vi "Modify Window Style.vi"(7 "Style Value":bool, 8 "GWL_EXStyle Modify":T1(ring), 9 "GWL_EXStyle In":u32 format="%.0x", 10 "GWL_Style Modify":T2(ring), 11 "GWL_Style In":u32 format="%.0x") -> (1 "GWL_EXStyle Out":u32 format="%.0x", 3 "GWL_Style Out":u32 format="%.0x")   [LabVIEW 2011]
doc: "This VI will modify the GWL_Style or GWL_EXStyle based on the value and key to modify."
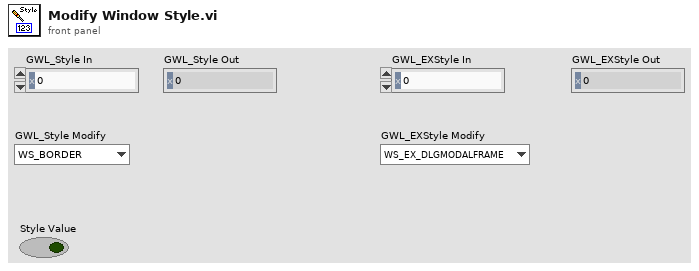
[diagram p1: front panel]
types:
  T1 = enum16{"WS_EX_DLGMODALFRAME", "WS_EX_NOPARENTNOTIFY", "WS_EX_TOPMOST", "WS_EX_ACCEPTFILES", "WS_EX_TRANSPARENT", "WS_EX_MDICHILD", "WS_EX_TOOLWINDOW", "WS_EX_WINDOWEDGE", "WS_EX_CLIENTEDGE", "WS_EX_CONTEXTHELP", "WS_EX_RIGHT", "WS_EX_LEFT", "WS_EX_RTLREADING", "WS_EX_LEFTSCROLLBAR", "WS_EX_CONTROLPARENT", "WS_EX_STATICEDGE", "WS_EX_APPWINDOW"}
  T2 = enum16{"WS_BORDER", "WS_CAPTION", "WS_CHILD", "WS_CLIPCHILDREN", "WS_CLIPSIBLINGS", "WS_DISABLED", "WS_DLGFRAME", "WS_HSCROLL", "WS_MAXIMIZE", "WS_MAXIMIZEBOX", "WS_MINIMIZE", "WS_MINIMIZEBOX", "WS_OVERLAPPED", "WS_POPUP", "WS_SYSMENU", "WS_THICKFRAME", "WS_VISIBLE", "WS_VSCROLL"}
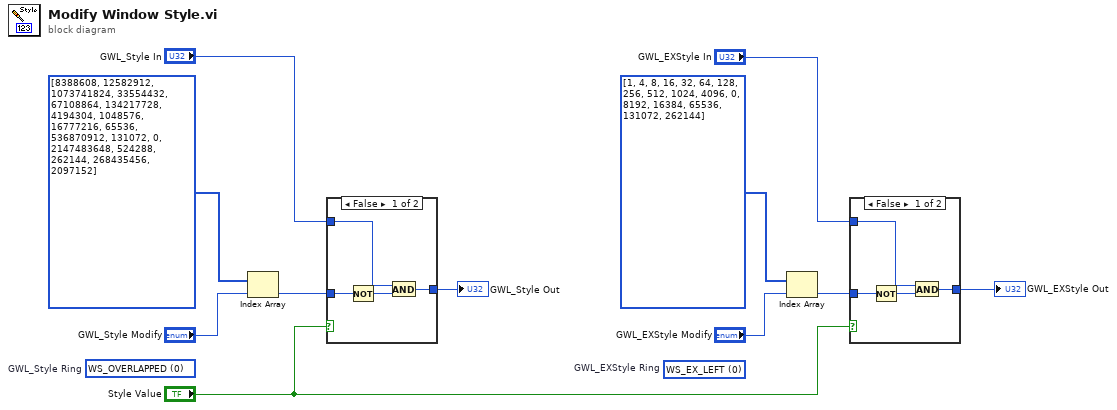
[diagram p0: block diagram]
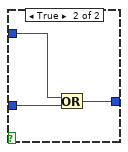
[diagram p2: hidden frame]
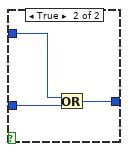
[diagram p3: hidden frame]
diagram:
  (unwired) u32 0 items=["WS_EX_DLGMODALFRAME"=1, "WS_EX_NOPARENTNOTIFY"=4, "WS_EX_TOPMOST"=8, "WS_EX_ACCEPTFILES"=16, "WS_EX_TRANSPARENT"=32, "WS_EX_MDICHILD"=64, "WS_EX_TOOLWINDOW"=128, "WS_EX_WINDOWEDGE"=256, "WS_EX_CLIENTEDGE"=512, "WS_EX_CONTEXTHELP"=1024, "WS_EX_RIGHT"=4096, "WS_EX_LEFT"=0, "WS_EX_RTLREADING"=8192, "WS_EX_LEFTSCROLLBAR"=16384, "WS_EX_CONTROLPARENT"=65536, "WS_EX_STATICEDGE"=131072, "WS_EX_APPWINDOW"=262144]  # GWL_EXStyle Ring
  (unwired) u32 0 items=["WS_BORDER"=8388608, "WS_CAPTION"=12582912, "WS_CHILD"=1073741824, "WS_CLIPCHILDREN"=33554432, "WS_CLIPSIBLINGS"=67108864, "WS_DISABLED"=134217728, "WS_DLGFRAME"=4194304, "WS_HSCROLL"=1048576, "WS_MAXIMIZE"=16777216, "WS_MAXIMIZEBOX"=65536, "WS_MINIMIZE"=536870912, "WS_MINIMIZEBOX"=131072, "WS_OVERLAPPED"=0, "WS_POPUP"=2147483648, "WS_SYSMENU"=524288, "WS_THICKFRAME"=262144, "WS_VISIBLE"=268435456, "WS_VSCROLL"=2097152]  # GWL_Style Ring
  n1 = Index Array(array=u32[] [8388608, 12582912, 1073741824, 33554432, 67108864, 134217728, 4194304, 1048576, 16777216, 65536, 536870912, 131072, 0, 2147483648, 524288, 262144, 268435456, 2097152] ("Array"), index="GWL_Style Modify") -> (element=w10:u32)
  n2 = case shown="False" "Style Value" {
    tunnel: w10 -> [w15 w18]
    tunnel: "GWL_Style In" -> [w14 w17]
    tunnel: [w13 w16] -> w8
    frame False {
      n3 = Not(x=w15) -> (.not. x?=w12:u32)
      n4 = And(x=w14, y=w12) -> (x .and. y?=w13:u32)
    }
    frame True {
      n5 = Or(x=w17, y=w18) -> (x .or. y?=w16:u32)
    }
  }
  "GWL_Style Out" <- w8
  n6 = Index Array(array=u32[] [1, 4, 8, 16, 32, 64, 128, 256, 512, 1024, 4096, 0, 8192, 16384, 65536, 131072, 262144] ("Array"), index="GWL_EXStyle Modify") -> (element=w6:u32)
  n7 = case shown="False" "Style Value" {
    tunnel: w6 -> [w22 w25]
    tunnel: "GWL_EXStyle In" -> [w21 w24]
    tunnel: [w20 w23] -> w1
    frame False {
      n8 = Not(x=w22) -> (.not. x?=w19:u32)
      n9 = And(x=w21, y=w19) -> (x .and. y?=w20:u32)
    }
    frame True {
      n10 = Or(x=w24, y=w25) -> (x .or. y?=w23:u32)
    }
  }
  "GWL_EXStyle Out" <- w1
